vi "AddElementToArray.vi"(0 "reference in":refnum<class "G#SubClass1.lvclass">, 5 "error in (no error)":errorcluster) -> (14 "reference out":refnum<class "G#SubClass1.lvclass">, 19 "error out":errorcluster)   [LabVIEW 2017, in "G#SubClass1.lvclass"]
uses:
  G#SubClass1.lvclass
  C:/Projects/GsharpGIT2017/Verification/TestCases/TestClasses/G#BaseClass1_class/G#BaseClass1.lvclass
  G#BaseClass1_class/G#BaseClass1.lvclass
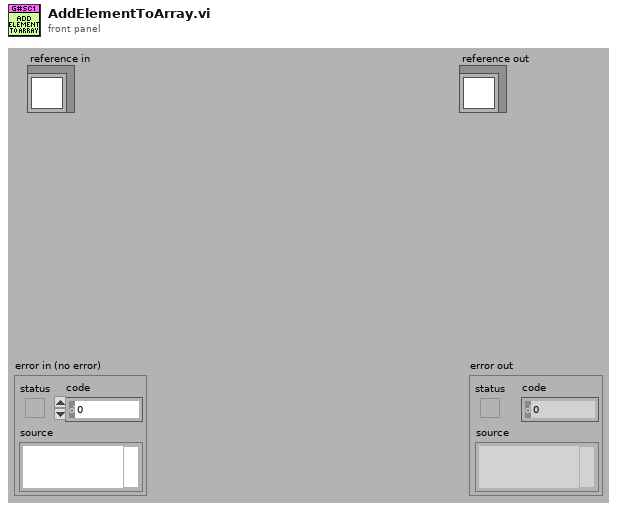
[diagram p1: front panel]
types:
  T1 = typedef "G#BaseClass1.lvclass/ObjectAttributesRef.ctl" = refnum<data-value>
  T2 = typedef "G#BaseClass1.lvclass/ObjectAttributes.ctl" = cluster{"Numeric":dbl, "Array":dbl[]}
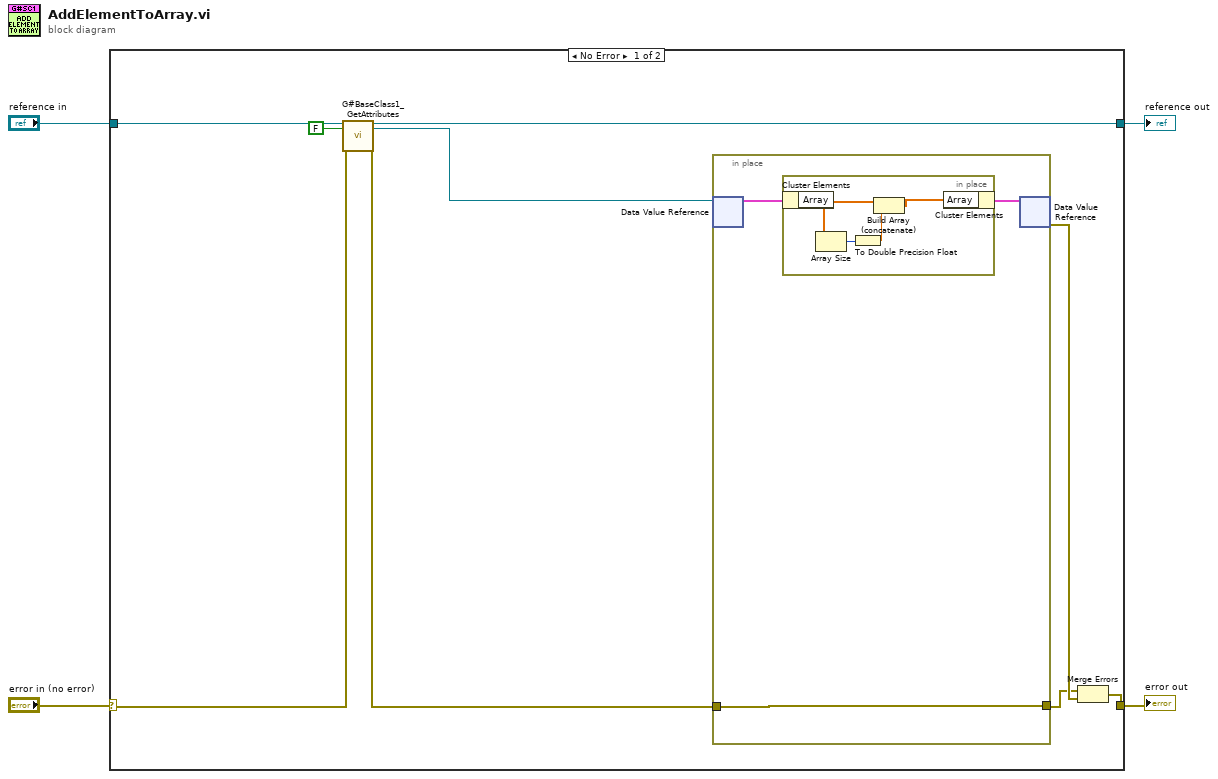
[diagram p0: block diagram]
diagram:
  n1 = case shown="No Error" "error in (no error)" {
    selector: "error in (no error)" -> [w8 w22]
    tunnel: [w13 w22] -> w3
    tunnel: [w9 w21] -> w1
    tunnel: "reference in" -> [w10 w21]
    frame No Error {
      n2 = call "G#BaseClass1_GetAttributes.vi"("reference in"=w10, "return data? (T)"=FALSE ("return data"), "error in (no error)"=w8) -> ("reference out"=w9:refnum<class "G#SubClass1.lvclass">, "attributes ref"=w5:T1, "error out"=w7:errorcluster)  [unwired: 13 in, 1 out]
      n3 = in-place {
        in-place-border: w7 -> [w14]
        in-place-border: [w14] -> w11
        n4 = in-place-dvr #1(w5) -> (w15:T2)  [unwired: 1 out]
        n5 = in-place {
          n6 = in-place-cluster #2(w15) -> ("Array"=w20:dbl[])
          n7 = Array Size(array=w20) -> (size(s)=w19:i32)
          n8 = To Double Precision Float(number=w19) -> (double precision float=w17:dbl)
          n9 = Build Array (concatenate)(w20, w17) -> (w18:dbl[])
          n10 = in-place-cluster #2("Array"=w18) -> (w16:T2)
        }
        n11 = in-place-dvr #1(w16) -> (w12:errorcluster)  [unwired: 1 out]
      }
      n12 = Merge Errors(w11, w12) -> (w13:errorcluster)
    }
    frame Error {
    }
  }
  "error out" <- w3
  "reference out" <- w1
